vi "Project Action.vi"(8 "error in (no error)":errorcluster, 11 "Toolbar Command":string) -> (0 "error out":errorcluster)   [LabVIEW 2016]
uses:
  DAQ-Display/PanelSplitToolkit/QueueManager.llb/Insert.vi
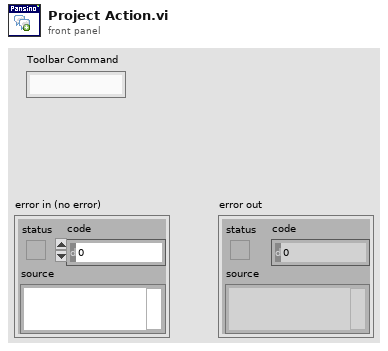
[diagram p1: front panel]
types:
  T1 = typedef "Global para Config.ctl" = cluster{"连续存储设置":cluster{"Save Mode":i32, "Sel Save Mode":i32, "FolderPath":path, "Filename":string, "Explation":string, "AutoPoint":i32, "Template":path}, "Latest Prj":path, "Tdms Ref*":refnum<k34>, "默认波形图个数":u8, "列表列数":u8}
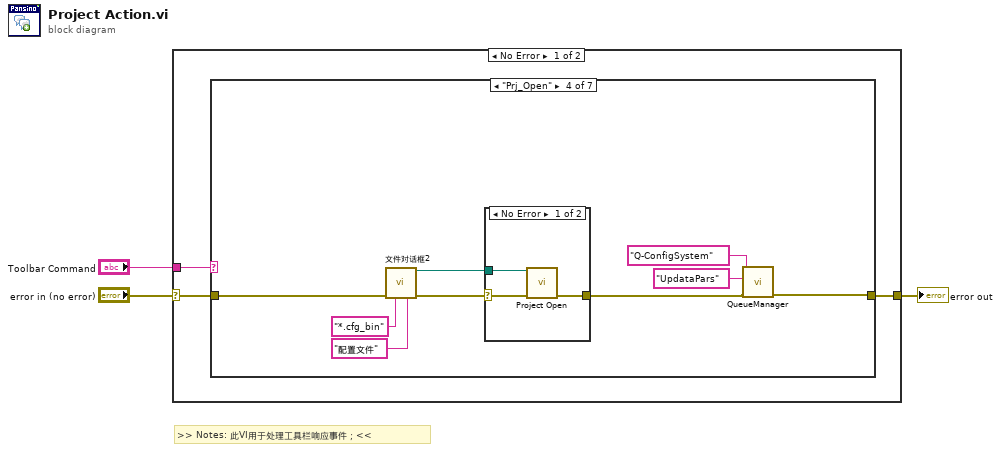
[diagram p0: block diagram]
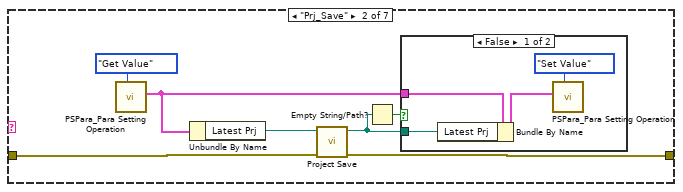
[diagram p3: hidden frame]
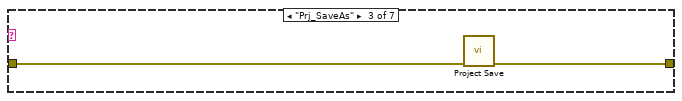
[diagram p5: hidden frame]
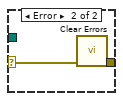
[diagram p6: hidden frame]
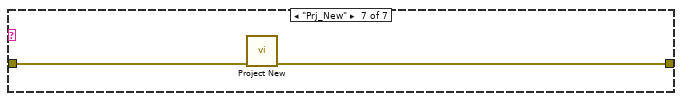
[diagram p9: hidden frame]
diagram:
  # ">> Notes: 此VI用于处理工具栏响应事件；<<"
  n1 = case shown="No Error" "error in (no error)" {
    selector: "error in (no error)" -> [w5 w39]
    tunnel: "Toolbar Command" -> [w6 _]
    tunnel: [w4 w39] -> w1
    frame No Error {
      n2 = case shown="\"Prj_Open\"" w6 {
        tunnel: w5 -> [w7 w14 w19 w25 w35 w36 w38]
        tunnel: [w7 w13 w20 w22 w35 w36 w37] -> w4
        frame "False", Default {
        }
        frame "Prj_Save" {
          n3 = call "PSPara_Para Setting Operation.vi"("Operation"=enum16{"Set Value", "Get Value", "Initialize"}."Get Value") -> ("_Para"=w10:T1)  [unwired: 9 in, 1 out]
          n4 = Unbundle By Name(w10) -> ("Latest Prj"=w11:path)
          n5 = call "Project Save.vi"("error in"=w14, "File Path"=w11) -> ("error out"=w13:errorcluster, "selected path"=w9:path)  [unwired: 8 in]
          n6 = Empty String/Path?(string/path=w9) -> (empty?=w8:bool)
          n7 = case shown="False" w8 {
            tunnel: w10 -> [w17 _]
            tunnel: w9 -> [w15 _]
            frame False {
              n8 = Bundle By Name(cluster=w17, "Latest Prj"=w15) -> (w16:T1)
              n9 = call "PSPara_Para Setting Operation.vi"("Operation"=enum16{"Set Value", "Get Value", "Initialize"}."Set Value", "_Para"=w16) -> ()  [unwired: 8 in, 2 out]
            }
            frame True {
            }
          }
        }
        frame "Prj_SaveAs" {
          n10 = call "Project Save.vi"("error in"=w19) -> ("error out"=w20:errorcluster)  [unwired: 9 in, 1 out]
        }
        frame "Prj_Open" {
          n11 = call "文件对话框2"("error in"=w25, "pattern (all files)"="*.cfg_bin", "pattern label"="配置文件") -> ("selected path"=w28:path, "error out"=w29:errorcluster)  [unwired: 9 in, 2 out]
          n12 = case shown="No Error" w29 {
            selector: w29 -> [w32 w34]
            tunnel: [w31 w33] -> w23
            tunnel: w28 -> [w30 _]
            frame No Error {
              n13 = call "Project Open.vi"("error in"=w32, "File Path"=w30) -> ("error out"=w31:errorcluster)  [unwired: 9 in]
            }
            frame Error {
              n14 = call <vilib>:"Clear Errors.vi"("error in (no error)"=w34) -> ("error out"=w33:errorcluster)  [unwired: 5 in, 1 out]
            }
          }
          n15 = call-poly "QueueManager.vi"("error in"=w23, "Event"="UpdataPars", "QueueName"="Q-ConfigSystem") -> ("error out"=w22:errorcluster)  [unwired: 7 in, 1 out]
        }
        frame "About" {
        }
        frame "Help" {
        }
        frame "Prj_New" {
          n16 = call "Project New.vi"("error in"=w38) -> ("error out"=w37:errorcluster)  [unwired: 10 in]
        }
      }
    }
    frame Error {
    }
  }
  "error out" <- w1
